vi "Get controls mapping for cluster.vi"(8 "error in (no error)":errorcluster, 11 "Ctl Refnum":refnum<vi>) -> (0 "error out":errorcluster, 1 "Mapping array":i32[](array[numeric]), 2 "Boolean labels array":string[](array[string]), 3 "Controls[]":refnum<vi>[](array[refnum]))   [LabVIEW 2015]
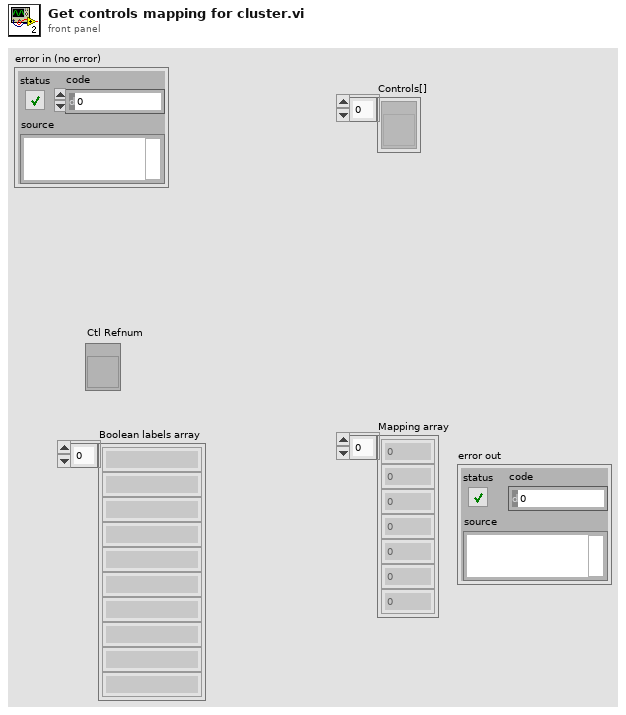
[diagram p1: front panel]
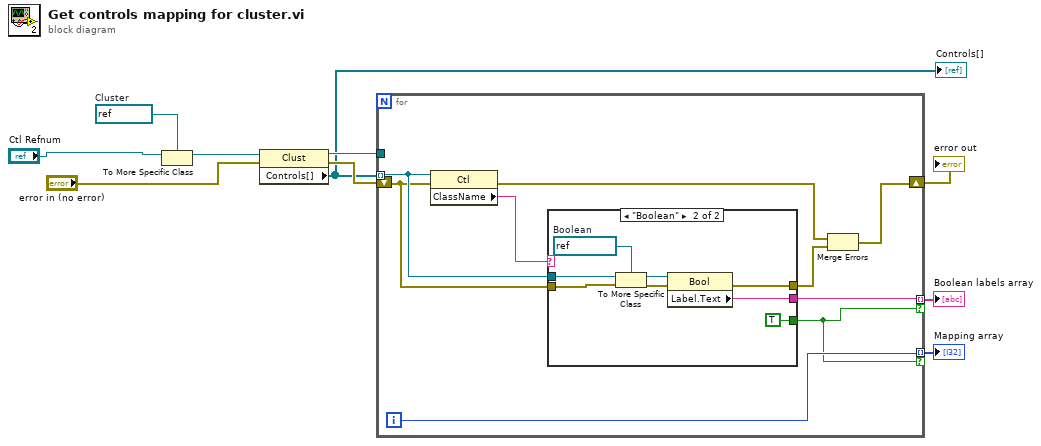
[diagram p0: block diagram]
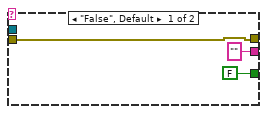
[diagram p2: hidden frame]
diagram:
  w3 = refnum<vi> refnum  # Cluster
  n1 = To More Specific Class(target class=w3, reference="Ctl Refnum") -> (specific class reference=w4:refnum<vi>)  [unwired: 1 in, 1 out]
  n2 = property class="Clust"(reference=w4, error in="error in (no error)") -> (reference out=w10:refnum<vi>, error out=w8:errorcluster, "Controls[]"=w7:refnum<vi>[])
  "Controls[]" <- w7
  n3 = for {
    tunnel: w10 -> [_]
    tunnel: w7 -> [w18] mode=indexing
    shift-right: [w11] -> w2
    shift-left: w8 -> [w17]
    tunnel: [w16] -> w6 mode=indexing if=w14
    tunnel: [w15] -> w5 mode=indexing if=w14
    i -> [w15]
    n4 = property class="Ctl"(reference=w18, error in=w17) -> (error out=w12:errorcluster, "ClassName"=w19:string)  [unwired: 1 out]
    n5 = case shown="\"Boolean\"" w19 {
      tunnel: w18 -> [_ w30]
      tunnel: w17 -> [w20 w29]
      tunnel: ["" ("Label.Text") w25] -> w16
      tunnel: [FALSE TRUE] -> w14
      tunnel: [w20 w23] -> w13
      frame "False", Default {
      }
      frame "Boolean" {
        w28 = refnum<vi> refnum  # Boolean
        n6 = To More Specific Class(target class=w28, reference=w30, error in=w29) -> (specific class reference=w27:refnum<vi>, error out=w26:errorcluster)
        n7 = property class="Bool"(reference=w27, error in=w26) -> (error out=w23:errorcluster, "Label.Text"=w25:string)  [unwired: 1 out]
      }
    }
    n8 = Merge Errors(w12, w13) -> (w11:errorcluster)
  }
  "Boolean labels array" <- w6
  "Mapping array" <- w5
  "error out" <- w2
